vi "user process.vi"(8 "error in":errorcluster, 11 "Parameters to process":T2) -> (0 "error out":errorcluster, 3 "Results from processing":T1)   [LabVIEW 2017, in "Tank Controller Logic runtime.lvclass"]
uses:
  Tank Controller Logic runtime.lvclass
  parameter user data.ctl
  result user data.ctl
  Tank State Machine Enum.ctl
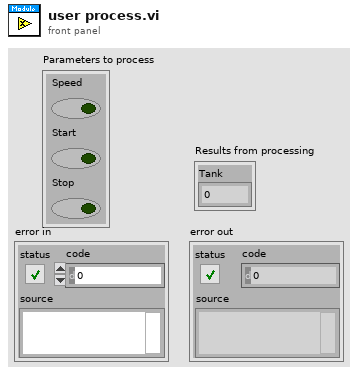
[diagram p1: front panel]
types:
  T1 = typedef "Tank Controller Logic runtime.lvclass/result user data.ctl" = cluster{"Tank":dbl}
  T2 = typedef "Tank Controller Logic runtime.lvclass/parameter user data.ctl" = cluster{"Speed":bool, "Start":bool, "Stop":bool}
  T3 = typedef "Tank State Machine Enum.ctl" = enum16{"idle", "fill", "tankFull"}
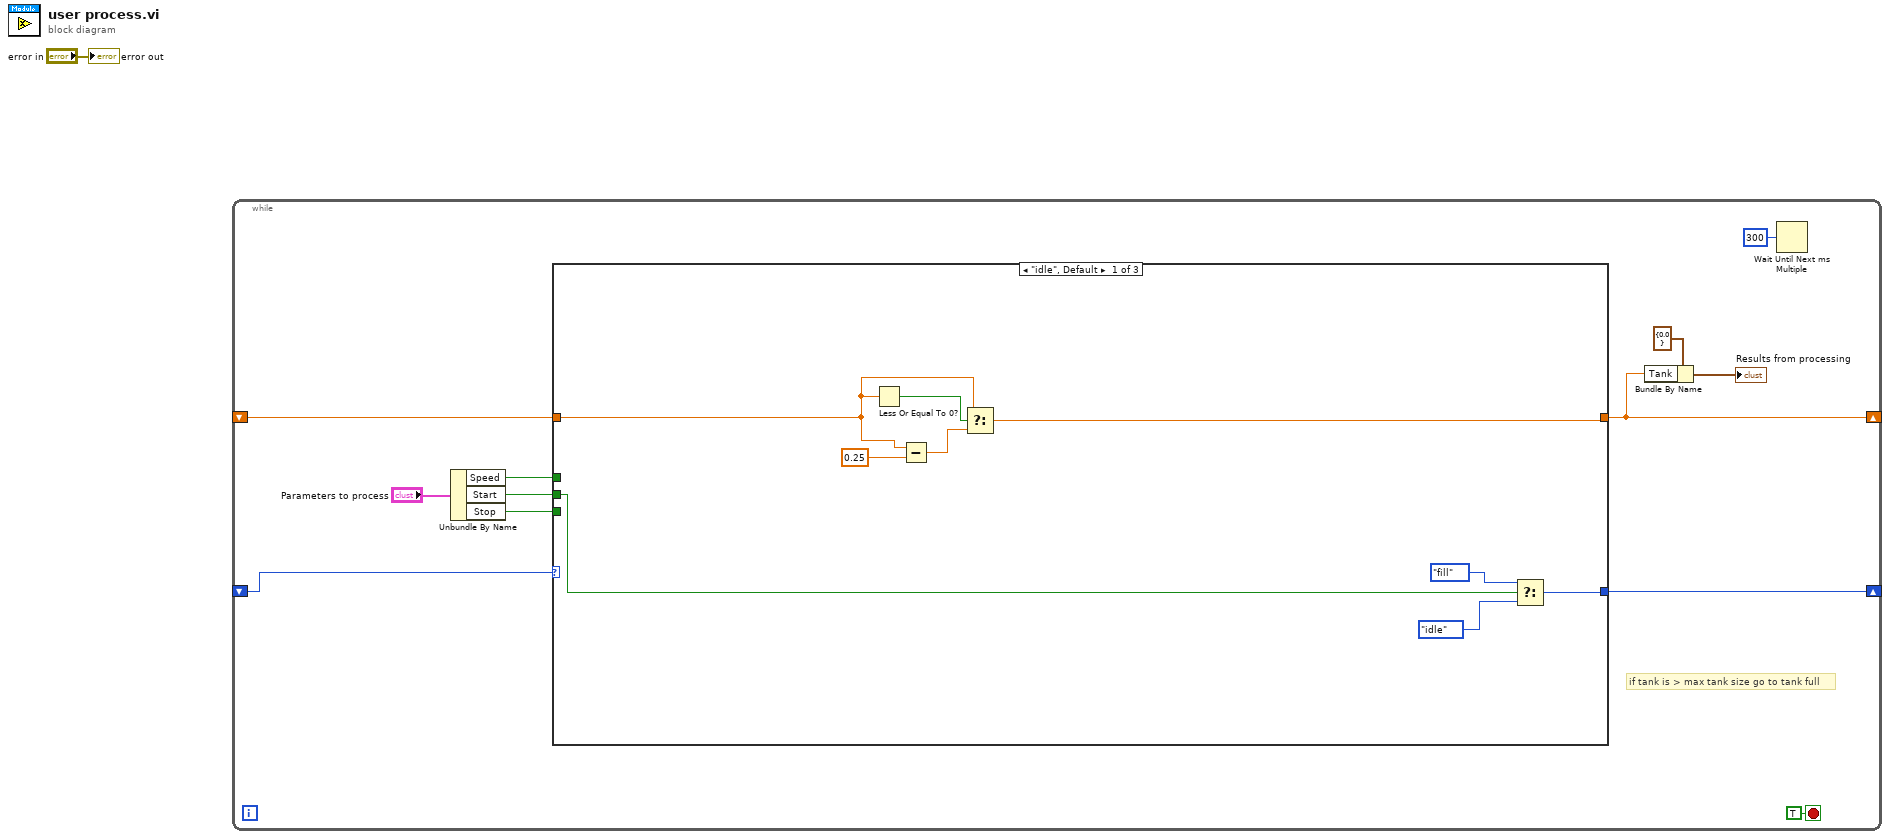
[diagram p0: block diagram]
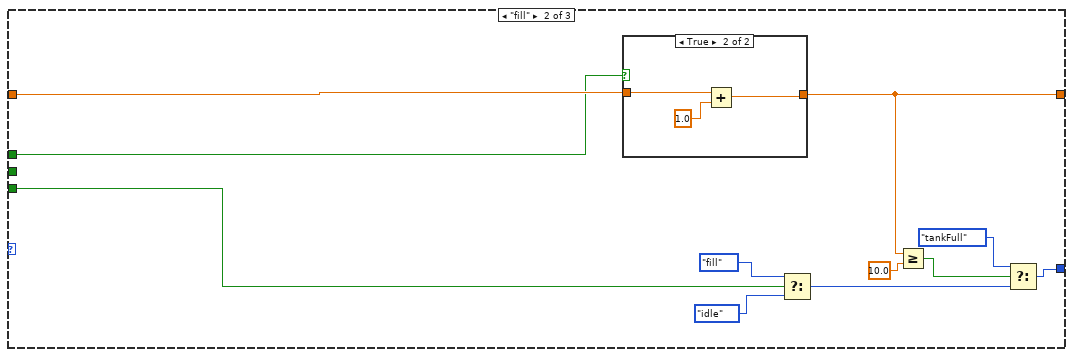
[diagram p2: hidden frame]
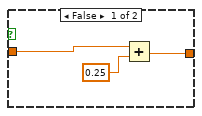
[diagram p3: hidden frame]
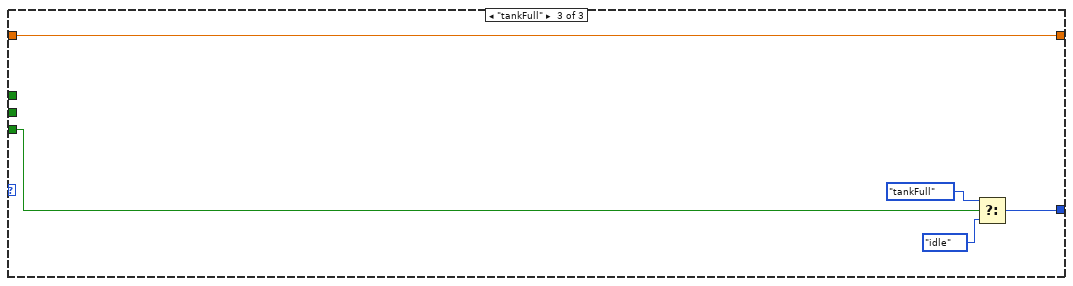
[diagram p4: hidden frame]
diagram:
  n1 = while {
    shift-right: [w9] -> _
    shift-left: _ -> [w12]
    shift-right: [w2] -> _
    shift-left: _ -> [w10]
    stop <- TRUE ("stop") stop-if-true
    # "if tank is > max tank size go to tank full"
    n2 = Unbundle By Name("Parameters to process") -> ("Speed"=w5:bool, "Start"=w4:bool, "Stop"=w3:bool)
    n3 = case shown="\"idle\", Default" w12 {
      tunnel: w10 -> [w15 w25 w44]
      tunnel: [w17 w31 w44] -> w2
      tunnel: [w19 w27 w41] -> w9
      tunnel: w5 -> [_ w24 _]
      tunnel: w4 -> [w14 _ _]
      tunnel: w3 -> [_ w23 w40]
      frame "idle", Default {
        n4 = Less Or Equal To 0?(x=w15) -> (x <= 0?=w16:bool)
        n5 = Subtract(x=w15, y=0.25) -> (x-y=w18:dbl)
        n6 = Select(t=w15, s=w16, f=w18) -> (s? t:f=w17:dbl)
        n7 = Select(t=Tank_State_Machine_Enum."fill", s=w14, f=Tank_State_Machine_Enum."idle") -> (s? t:f=w19:T3)
      }
      frame "fill" {
        n8 = case shown="True" w24 {
          tunnel: [w35 w38] -> w31
          tunnel: w25 -> [w34 w37]
          frame False {
            n9 = Add(x=w34, y=0.25) -> (x+y=w35:dbl)
          }
          frame True {
            n10 = Add(x=w37, y=1.0) -> (x+y=w38:dbl)
          }
        }
        n11 = Select(t=Tank_State_Machine_Enum."fill", s=w23, f=Tank_State_Machine_Enum."idle") -> (s? t:f=w26:T3)
        n12 = Greater Or Equal?(x=w31, y=10.0) -> (x >= y?=w30:bool)
        n13 = Select(t=Tank_State_Machine_Enum."tankFull", s=w30, f=w26) -> (s? t:f=w27:T3)
      }
      frame "tankFull" {
        n14 = Select(t=Tank_State_Machine_Enum."tankFull", s=w40, f=Tank_State_Machine_Enum."idle") -> (s? t:f=w41:T3)
      }
    }
    n15 = Bundle By Name(cluster=T1 {"Tank"=0.0} ("Results from processing"), "Tank"=w2) -> (→"Results from processing":T1)
    n16 = Wait Until Next ms Multiple(millisecond multiple=u32 300) -> ()  [unwired: 1 out]
  }
  "error out" <- "error in"
